vi "UHR-Fleezers Control (host) - Lorentz v5.vi"() -> ()   [LabVIEW 2014] (continued)
        n1320 = property on="Blue Laser ON" class="Bool (strict)"("Val(Sgnl)"="Blue Laser ON/OFF") -> ()  [unwired: 2 in, 2 out]
        n1321 = property on="Green Laser ON" class="Bool (strict)"("Val(Sgnl)"="Green Laser ON/OFF") -> ()  [unwired: 2 in, 2 out]
      }
      event "Laser interlacing mode", "Green Laser ON", "Red Laser ON", "Blue Laser ON": Value Change {
        n1322 = event-data() -> ()  [unwired: 7 out]
        n1323 = local write "Green Laser ON/OFF"("Green Laser ON") -> ()
        n1324 = local write "Blue Laser ON/OFF"("Blue Laser ON") -> ()
        n1325 = local write "Red Laser ON/OFF"("Red Laser ON") -> ()
        n1326 = case shown="False" "Green Laser ON" {
          tunnel: "Laser interlacing mode" -> [_ w2077]
          tunnel: [enum32{"Laser ON", "Laser OFF", "Interlace"}."Laser OFF" ("Green laser mode") w2077] -> w2053
          tunnel: [FALSE w2073] -> w2052
          frame False {
          }
          frame True {
            n1327 = local read "Green FB On/Off"() -> (w2074:bool)
            n1328 = Equal?(x=w2077, y=enum32{"Laser ON", "Laser OFF", "Interlace"}."Interlace") -> (x = y?=w2075:bool)
            n1329 = And(x=w2075, y=w2074) -> (x .and. y?=w2073:bool)
          }
        }
        n1330 = case shown="True" "Red Laser ON" {
          tunnel: "Laser interlacing mode" -> [_ w2070]
          tunnel: [enum32{"Laser ON", "Laser OFF", "Interlace"}."Laser OFF" ("Green laser mode") w2070] -> w2049
          tunnel: [FALSE w2066] -> w2048
          frame False {
          }
          frame True {
            n1331 = local read "Red FB On/Off"() -> (w2067:bool)
            n1332 = Equal?(x=w2070, y=enum32{"Laser ON", "Laser OFF", "Interlace"}."Interlace") -> (x = y?=w2068:bool)
            n1333 = And(x=w2068, y=w2067) -> (x .and. y?=w2066:bool)
          }
        }
        n1334 = case shown="True" "Blue Laser ON" {
          tunnel: "Laser interlacing mode" -> [_ w2061]
          tunnel: [enum32{"Laser ON", "Laser OFF", "Interlace"}."Laser OFF" ("Green laser mode") w2061] -> w2045
          tunnel: [FALSE w2059] -> w2044
          frame False {
          }
          frame True {
            n1335 = local read "Blue FB On/Off"() -> (w2060:bool)
            n1336 = Equal?(x=w2061, y=enum32{"Laser ON", "Laser OFF", "Interlace"}."Interlace") -> (x = y?=w2062:bool)
            n1337 = And(x=w2062, y=w2060) -> (x .and. y?=w2059:bool)
          }
        }
        n1338 = xnode "Read/Write Control"("FPGA VI Reference In"=w2043, "Operating Mode"=w2053, "Operating Mode 2"=w2053, "Green FB On/Off"=w2052, "Red Laser Operating Mode"=w2049, "RI Operating Mode 2"=w2049, "Red FB On/Off"=w2048, "BI Operating Mode (AO)"=w2045, "Blue Laser Operating Mode (D)"=w2045, "Blue FB On/Off"=w2044) -> ("error out"=w2054:errorcluster)  [unwired: 1 in, 1 out]
        n1339 = local read "Red FB On/Off"() -> (w2026:bool)
        n1340 = local read "Green FB On/Off"() -> (w2028:bool)
        n1341 = local read "Green Laser ON"() -> (w2027:bool)
        n1342 = local read "Red Laser ON"() -> (w2025:bool)
        n1343 = And(x=w2026, y=w2025) -> (x .and. y?=w2031:bool)
        n1344 = And(x=w2028, y=w2027) -> (x .and. y?=w2037:bool)
        n1345 = local read "Red laser intensity (V)"() -> (w2030:dbl)
        n1346 = local read "Red FB Setpoint (mV)"() -> (w2029:dbl)
        n1347 = local read "Green FB Setpoint (mV)"() -> (w2040:dbl)
        n1348 = local read "Green laser intensity (V)"() -> (w2042:dbl)
        n1349 = Multiply(x=w2030, y=1000.0) -> (x*y=w2034:dbl)
        n1350 = Subtract(x=w2029, y=5.0) -> (x-y=w2033:dbl)
        n1351 = Multiply(x=w2042, y=1000.0) -> (x*y=w2039:dbl)
        n1352 = Subtract(x=w2040, y=5.0) -> (x-y=w2038:dbl)
        n1353 = Less Or Equal?(x=w2034, y=w2033) -> (x <= y?=w2032:bool)
        n1354 = Less Or Equal?(x=w2039, y=w2038) -> (x <= y?=w2036:bool)
        n1355 = And(x=w2031, y=w2032) -> (x .and. y?=w2021:bool)
        n1356 = And(x=w2037, y=w2036) -> (x .and. y?=w2022:bool)
        n1357 = Or(x=w2022, y=w2021) -> (x .or. y?=w2020:bool)
        n1358 = case shown="True" w2020 {
          frame False {
            n1359 = local write "Laser Intensity Low (bugs to fix)"(FALSE ("Laser Intensity Low")) -> ()
          }
          frame True {
            n1360 = local write "Laser Intensity Low (bugs to fix)"(TRUE ("Laser Intensity Low")) -> ()
          }
        }
      }
      event "Invert laser interlacing": Value Change {
        n1361 = event-data() -> ()  [unwired: 7 out]
        n1362 = xnode "Read/Write Control"("FPGA VI Reference In"=w2078, "Invert GI"="Invert laser interlacing", "Invert GI 2"="Invert laser interlacing", "Invert RI"="Invert laser interlacing", "Invert RI 2"="Invert laser interlacing", "Invert BI (AO)"="Invert laser interlacing", "Invert BI (D)"="Invert laser interlacing") -> ("error out"=w2080:errorcluster)  [unwired: 1 in, 1 out]
      }
      event "Green FB Setpoint (mV)", "Green FB Gains", "Green FB On/Off", "Green Intensity % (FB OFF)", "Green int current ON count adj": Value Change {
        n1363 = event-data() -> ()  [unwired: 7 out]
        n1364 = local read "Green FB Setpoint (mV)"() -> (w2100:dbl)
        n1365 = Multiply(x=w2100, y=3.2767) -> (x*y=w2099:dbl)
        n1366 = local read "Green Intensity % (FB OFF)"() -> (w2103:dbl)
        n1367 = Multiply(x=w2103, y=655.35) -> (x*y=w2104:dbl)
        n1368 = To Unsigned Word Integer(number=w2104) -> (unsigned 16bit integer=w2102:u16)
        n1369 = local read "Green int current ON count adj"() -> (w2106:u32)
        n1370 = local read "Laser interlacing mode"() -> (w2097:enum32{"Laser ON", "Laser OFF", "Interlace"})
        n1371 = local read "Green FB Gains"() -> (w2094:T14)
        n1372 = local read "Green Laser ON"() -> (w2098:bool)
        n1373 = local read "Green FB On/Off"() -> (w2107:bool)
        n1374 = Equal?(x=w2097, y=enum32{"Laser ON", "Laser OFF", "Interlace"}."Interlace") -> (x = y?=w2095:bool)
        n1375 = Unbundle By Name(w2094) -> ("proportional gain (Kc)"=w2093:i16, "integral gain (Kc*Ts/Ti)"=w2092:i16, "derivative gain (Kc*Td/Ts)"=w2091:i16)
        n1376 = Compound Arithmetic op=AND(w2095, w2107, w2098) -> (w2081:bool)
        n1377 = local read "Green FB Setpoint (mV)"() -> (w2085:dbl)
        n1378 = local read "Green laser intensity (V)"() -> (w2088:dbl)
        n1379 = xnode "Read/Write Control"("FPGA VI Reference In"=w2090, "Green FB Setpoint"=w2099, "Green FB On/Off"=w2081, "Current Out"=w2102, "Green int current ON count adj"=w2106, "P3"=w2093, "I3"=w2092, "D3"=w2091) -> ("error out"=w2108:errorcluster)  [unwired: 1 in, 1 out]
        n1380 = Multiply(x=w2088, y=1000.0) -> (x*y=w2084:dbl)
        n1381 = Subtract(x=w2085, y=5.0) -> (x-y=w2083:dbl)
        n1382 = Less Or Equal?(x=w2084, y=w2083) -> (x <= y?=w2082:bool)
        n1383 = And(x=w2081, y=w2082) -> (x .and. y?=w2089:bool)
        n1384 = case shown="True" w2089 {
          frame False {
            n1385 = local write "Laser Intensity Low (bugs to fix)"(FALSE ("Laser Intensity Low")) -> ()
          }
          frame True {
            n1386 = local write "Laser Intensity Low (bugs to fix)"(TRUE ("Laser Intensity Low")) -> ()
          }
        }
      }
      event "Blue FB Setpoint (mV)", "Blue FB Gains", "Blue FB On/Off", "Blue Intensity % (FB OFF)", "Blue int AO ON count adjust": Value Change {
        # "Triggers blue laser serial command"
        # "16 bit analog out"
        n1387 = event-data() -> ()  [unwired: 7 out]
        n1388 = Multiply(x="Blue FB Setpoint (mV)", y=3.2767) -> (x*y=w2128:dbl)
        n1389 = Multiply(x="Blue Intensity % (FB OFF)", y=0.8) -> (x*y=w2111:dbl)
        n1390 = Number To Decimal String(number=w2111) -> (decimal integer string=w2112:string)  [unwired: 1 in]
        n1391 = Multiply(x="Blue Intensity % (FB OFF)", y=655.35) -> (x*y=w2131:dbl)
        n1392 = local write "Blue Laser Power (mW)\n(Constant Power Mode)"(w2112) -> ()
        n1393 = To Unsigned Word Integer(number=w2131) -> (unsigned 16bit integer=w2130:u16)
        n1394 = local read "Laser interlacing mode"() -> (w2126:enum32{"Laser ON", "Laser OFF", "Interlace"})
        n1395 = Unbundle By Name("Blue FB Gains") -> ("proportional gain (Kc)"=w2123:i16, "integral gain (Kc*Ts/Ti)"=w2122:i16, "derivative gain (Kc*Td/Ts)"=w2121:i16)
        n1396 = local read "Blue Laser ON"() -> (w2116:bool)
        n1397 = Equal?(x=w2126, y=enum32{"Laser ON", "Laser OFF", "Interlace"}."Interlace") -> (x = y?=w2124:bool)
        n1398 = Compound Arithmetic op=AND(w2124, "Blue FB On/Off", w2116) -> (w2127:bool)
        n1399 = xnode "Read/Write Control"("FPGA VI Reference In"=w2115, "Blue FB Setpoint"=w2128, "Blue FB On/Off"=w2127, "BI Current Out"=w2130, "Blue current ON count adj (AO)"="Blue int AO ON count adjust", "P5"=w2123, "I5"=w2122, "D5"=w2121) -> ("error out"=w2133:errorcluster)  [unwired: 1 in, 1 out]
      }
      event "Red FB Setpoint (mV)", "Red FB Gains", "Red FB On/Off", "Red Intensity % (FB OFF)": Value Change {
        n1400 = event-data() -> ()  [unwired: 7 out]
        n1401 = local read "Red FB Setpoint (mV)"() -> (w2154:dbl)
        n1402 = Multiply(x=w2154, y=3.2767) -> (x*y=w2153:dbl)
        n1403 = local read "Red Intensity % (FB OFF)"() -> (w2144:dbl)
        n1404 = Multiply(x=w2144, y=655.35) -> (x*y=w2157:dbl)
        n1405 = To Unsigned Word Integer(number=w2157) -> (unsigned 16bit integer=w2156:u16)
        n1406 = local read "Laser interlacing mode"() -> (w2151:enum32{"Laser ON", "Laser OFF", "Interlace"})
        n1407 = local read "Red FB Gains"() -> (w2148:T14)
        n1408 = local read "Red Laser ON"() -> (w2152:bool)
        n1409 = local read "Red FB On/Off"() -> (w2159:bool)
        n1410 = Equal?(x=w2151, y=enum32{"Laser ON", "Laser OFF", "Interlace"}."Interlace") -> (x = y?=w2149:bool)
        n1411 = Unbundle By Name(w2148) -> ("proportional gain (Kc)"=w2147:i16, "integral gain (Kc*Ts/Ti)"=w2146:i16, "derivative gain (Kc*Td/Ts)"=w2145:i16)
        n1412 = Compound Arithmetic op=AND(w2149, w2159, w2152) -> (w2136:bool)
        n1413 = local read "Red laser intensity (V)"() -> (w2135:dbl)
        n1414 = local read "Red FB Setpoint (mV)"() -> (w2134:dbl)
        n1415 = xnode "Read/Write Control"("FPGA VI Reference In"=w2143, "Red FB Setpoint"=w2153, "Red FB On/Off"=w2136, "RI Current Out"=w2156, "P4"=w2147, "I4"=w2146, "D4"=w2145) -> ("error out"=w2160:errorcluster)  [unwired: 1 in, 1 out]
        n1416 = Multiply(x=w2135, y=1000.0) -> (x*y=w2140:dbl)
        n1417 = Subtract(x=w2134, y=5.0) -> (x-y=w2139:dbl)
        n1418 = Less Or Equal?(x=w2140, y=w2139) -> (x <= y?=w2138:bool)
        n1419 = And(x=w2136, y=w2138) -> (x .and. y?=w2137:bool)
        n1420 = case shown="False" w2137 {
          frame False {
            n1421 = local write "Laser Intensity Low (bugs to fix)"(FALSE ("Laser Intensity Low")) -> ()
          }
          frame True {
            n1422 = local write "Laser Intensity Low (bugs to fix)"(TRUE ("Laser Intensity Low")) -> ()
          }
        }
      }
      event "+ phase (APD 1 Gate)", "- phase (APD 1 Gate)", "+ phase (APD 2 Gate)", "- phase (APD 2 Gate)", "+ phase (APD 3 Gate)", "- phase (APD 3 Gate)", "+ phase (APD Acq)", "- phase (APD Acq)": Value Change {
        n1423 = event-data() -> ()  [unwired: 7 out]
        n1424 = local read "Phase Adj. (APD 1 Gate)"() -> (w2183:i16)
        n1425 = Or(x="- phase (APD 1 Gate)", y="+ phase (APD 1 Gate)") -> (x .or. y?=w2185:bool)
        n1426 = Negate(x=w2183) -> (-x=w2190:i16)
        n1427 = Select(t=w2190, s="+ phase (APD 1 Gate)", f=w2183) -> (s? t:f=w2189:i16)
        n1428 = local read "Phase Adj. (APD 2 Gate)"() -> (w2180:i16)
        n1429 = Or(x="- phase (APD 2 Gate)", y="+ phase (APD 2 Gate)") -> (x .or. y?=w2178:bool)
        n1430 = Negate(x=w2180) -> (-x=w2182:i16)
        n1431 = Select(t=w2182, s="+ phase (APD 2 Gate)", f=w2180) -> (s? t:f=w2179:i16)
        n1432 = Negate(x="Phase Adj. (APD 3 Gate)") -> (-x=w2177:i16)
        n1433 = Or(x="- phase (APD 3 Gate)", y="+ phase (APD 3 Gate)") -> (x .or. y?=w2173:bool)
        n1434 = Select(t=w2177, s="+ phase (APD 3 Gate)", f="Phase Adj. (APD 3 Gate)") -> (s? t:f=w2174:i16)
        n1435 = local read "Phase Adj. (APD Acq)"() -> (w2171:i16)
        n1436 = Or(x="- phase (APD Acq)", y="+ phase (APD Acq)") -> (x .or. y?=w2169:bool)
        n1437 = Negate(x=w2171) -> (-x=w2172:i16)
        n1438 = Select(t=w2172, s="+ phase (APD Acq)", f=w2171) -> (s? t:f=w2170:i16)
        n1439 = xnode "Read/Write Control"("FPGA VI Reference In"=w2163, "Phase count adjustment (APD 1 Gate)"=w2189, "Phase count adjustment (APD 2 Gate)"=w2179, "Phase count adjustment (APD 3 Gate)"=w2174, "Phase Count Adjustment (APD Acq)"=w2170) -> ("FPGA VI Reference Out"=w2187:T35, "error out"=w2188:errorcluster)  [unwired: 1 in]
        n1440 = xnode "Read/Write Control"("FPGA VI Reference In"=w2187, "error in"=w2188, "+ phase (APD 1 Gate)"=w2185, "+ phase (APD 2 Gate)"=w2178, "+ phase (APD 3 Gate)"=w2173, "+ phase (APD Acq)"=w2169) -> ("error out"=w2186:errorcluster)  [unwired: 1 out]
      }
      event "Invert APD Gate", "APD Gate ON Count", "APD Gate OFF Count", "APD Gate", "APD Integration Time (s)", "APD AO Scale Factor", "Duty Frequency (ON 1/N cycles)", "Interlace ON count", "Interlace OFF count": Value Change {
        n1441 = event-data() -> ()  [unwired: 7 out]
        n1442 = Add(x="Interlace ON count", y="Interlace OFF count") -> (x+y=w2197:u16)
        n1443 = Add(x="APD Gate ON Count", y="APD Gate OFF Count") -> (x+y=w2208:u16)
        n1444 = Multiply(x="Duty Frequency (ON 1/N cycles)", y=w2197) -> (x*y=w2193:u16)
        "Green AI Count" <- w2193
        "Red AI Count" <- w2193
        "Blue AI Count" <- w2193
        n1445 = Subtract(x=w2193, y="Interlace ON count") -> (x-y=w2196:u16)
        n1446 = Multiply(x=w2208, y="Duty Frequency (ON 1/N cycles)") -> (x*y=w2207:u16)
        n1447 = Subtract(x=w2207, y="APD Gate ON Count") -> (x-y=w2206:u16)
        n1448 = local read "DMA Update Period (s)"() -> (w2209:dbl)
        n1449 = Multiply(x="APD Integration Time (s)", y=40000000.0) -> (x*y=w2213:dbl)
        n1450 = Reciprocal(x="APD Integration Time (s)") -> (1/x=→"APD Acq Rate (Hz)":dbl)
        n1451 = To Unsigned Long Integer(number=w2213) -> (unsigned 32bit integer=w2199:u32)
        "APD Int. Count" <- w2199
        n1452 = local read "Number of APDs"() -> (w2192:u8)
        n1453 = Divide(x=w2209, y="APD Integration Time (s)") -> (x/y=w2211:dbl)
        n1454 = Multiply(x=w2192, y=w2211) -> (x*y=w2210:dbl)
        n1455 = local write "APD Samples/FIFO Acq."(w2211) -> ()
        n1456 = local write "APD Elements/DMA read"(w2210) -> ()
        n1457 = xnode "Read/Write Control"("FPGA VI Reference In"=w2191, "Invert APD Gate"="Invert APD Gate", "APD Gate ON Count"="APD Gate ON Count", "APD Gate OFF Count"=w2206, "APD Acq Rate Count"=w2199, "APD Gate Operating Mode"="APD Gate", "APD AO scale factor"="APD AO Scale Factor", "Green interlace ON count"="Interlace ON count", "Green interlace OFF count"=w2196, "Green interlace ON count 2"="Interlace ON count", "Green interlace OFF count 2"=w2196, "Green FB Count"=w2193, "Red interlace ON count"="Interlace ON count", "Red interlace OFF count"="Interlace OFF count", "Blue ON count (AO)"="Interlace ON count", "Blue OFF count (AO)"="Interlace OFF count", "Blue interlace OFF count (D)"="Interlace OFF count", "Blue interlace ON count (D)"="Interlace ON count") -> ("error out"=w2215:errorcluster)  [unwired: 1 in, 1 out]
      }
      event "Neg. TTrig FPGA": Value Change {
        n1458 = event-data() -> ()  [unwired: 7 out]
        n1459 = xnode "Read/Write Control"("FPGA VI Reference In"=w2216, "TTrig Negate Pos"="Neg. TTrig FPGA") -> ()  [unwired: 1 in, 2 out]
      }
      event "Test ttrig": Value Change {
        n1460 = event-data() -> ()  [unwired: 7 out]
        n1461 = xnode "Read/Write Control"("FPGA VI Reference In"=w2218, "TTrig?"=TRUE) -> ("error out"=w2220:errorcluster)  [unwired: 1 in, 1 out]
      }
      event "Number of F/B Scans (AOD)", "Scan Speed (nm/s)", "Scan BD", "Initial delta (MHz)", "Step Size (nm)", "Scan Range (nm)": Value Change {
        w2284 = 123.0  # AOM cal (nm/MHz)
        n1462 = event-data() -> ()  [unwired: 7 out]
        n1463 = local read "BD 1 Frequency 1 (MHz)"() -> (w2267:dbl)
        n1464 = local read "AOM X Cal (nm/MHz)"() -> (w2259:dbl)
        n1465 = local read "X RF Frequency Limits (MHz)"() -> (w2271:T23)
        n1466 = local read "Y RF Frequency Limits (MHz)"() -> (w2268:T23)
        n1467 = local read "BD 2 Frequency 1 (MHz)"() -> (w2273:dbl)
        n1468 = Negate(x="Scan Range (nm)") -> (-x=w2237:dbl)
        n1469 = Divide(x=w2237, y=w2259) -> (x/y=w2241:dbl)
        n1470 = Select(t=w2271, s="Scan BD", f=w2268) -> (s? t:f=w2270:T23)
        n1471 = Select(t=w2267, s="Scan BD", f=w2273) -> (s? t:f=w2272:dbl)
        n1472 = Unbundle By Name(w2270) -> ("Maximum"=w2279:dbl, "Minimum"=w2278:dbl)
        n1473 = Add(x=w2241, y=w2272) -> (x+y=w2276:dbl)
        n1474 = Divide(x=w2237, y="Step Size (nm)") -> (x/y=w2256:dbl)
        n1475 = Divide(x="Step Size (nm)", y=w2259) -> (x/y=w2265:dbl)
        n1476 = Absolute Value(x=w2256) -> (abs(x)=w2240:dbl)
        n1477 = Sign(1:w2237) -> (0:w2238:dbl)
        n1478 = In Range and Coerce(upper limit=w2279, x=w2276, lower limit=w2278) -> (coerced(x)=w2275:dbl, In Range?=w2277:bool)
        n1479 = To Unsigned Quad Integer(1:w2240) -> (0:w2255:u64)
        "Scan steps (AOD)" <- w2255
        n1480 = call "IR AOM freq to word.vi"("Frequency In (MHz)"=w2265) -> ("Frequency Word Out (double)"=w2262:dbl)
        n1481 = Multiply(x=w2238, y=w2262) -> (x*y=w2239:dbl)
        n1482 = Subtract(x=w2276, y=w2275) -> (x-y=w2274:dbl)
        n1483 = To Quad Integer(1:w2239) -> (0:w2261:i64)
        "Incr. int (AOD)" <- w2261
        n1484 = Subtract(x=w2241, y=w2274) -> (x-y=w2260:dbl)
        "Scan Range (MHz)" <- w2260
        n1485 = Select(t=w2241, s=w2277, f=w2260) -> (s? t:f=w2280:dbl)
        n1486 = Multiply(x=w2260, y=w2259) -> (x*y=w2258:dbl)
        n1487 = Decrement(x=w2255) -> (x-1=w2308:u64)
        n1488 = Negate(x=w2258) -> (-x=w2254:dbl)
        n1489 = local write "Scan Range (nm)"(w2254) -> ()
        n1490 = Divide(x=w2280, y=w2308) -> (x/y=w2264:dbl)
        "Scan Increment (MHz)" <- w2264
        n1491 = call "IR AOM freq to word.vi"("Frequency In (MHz)"=w2264) -> ("Frequency Word Out (double)"=w2263:dbl)
        n1492 = Divide(x="Step Size (nm)", y="Scan Speed (nm/s)") -> (x/y=w2251:dbl)
        n1493 = To Quad Integer(1:w2263) -> ()  [unwired: 1 out]
        n1494 = local read "Number Interlace Sets"() -> (w2235:u8)
        n1495 = local read "AI Count (ticks)"() -> (w2236:u16)
        n1496 = local read "Total Counts (ticks)"() -> (w2234:u16)
        n1497 = local read "# Samples/trap"() -> (w2266:u32)
        n1498 = Multiply(x=w2236, y=w2235) -> (x*y=w2233:u16)
        n1499 = Divide(x=w2234, y=w2233) -> (x/y=w2232:dbl)
        n1500 = Select(t=w2267, s="Scan BD", f=w2273) -> (s? t:f=w2305:dbl)
        "Initial freq. (MHz)" <- w2305
        n1501 = Add(x=w2280, y=w2305) -> (x+y=→"Final freq. (MHz)":dbl)
        n1502 = Divide(x=w2234, y=40000000.0) -> (x/y=w2250:dbl)
        n1503 = Divide(x=w2251, y=w2250) -> (x/y=w2249:dbl)
        n1504 = To Unsigned Quad Integer(1:w2249) -> (0:w2224:u64)
        n1505 = Quotient & Remainder(x=w2224, y=u64 2) -> (x-y*floor(x/y)=w2228:u64)  [unwired: 1 out]
        n1506 = Equal?(x=w2228, y=u64 0) -> (x = y?=w2226:bool)
        n1507 = Decrement(x=w2224) -> (x-1=w2225:u64)
        n1508 = Select(t=w2224, s=w2226, f=w2225) -> (s? t:f=w2223:u64)
        "Cycles/step (AOD)" <- w2223
        n1509 = xnode "Read/Write Control"("FPGA VI Reference In"=w2222, "Scan steps"=w2255, "Number of scans"="Number of F/B Scans (AOD)", "Cycles per step"=w2223, "Scan freq.  increment"=w2261, "Scan BD"="Scan BD") -> ("error out"=w2314:errorcluster)  [unwired: 1 in, 1 out]
        n1510 = Multiply(x=w2255, y=w2223) -> (x*y=w2309:u64)
        n1511 = Multiply(x=w2309, y=u64 2) -> (x*y=w2231:u64)
        n1512 = Multiply(x=w2232, y=w2231) -> (x*y=w2230:dbl)
        "Data points/scan (f/b)" <- w2230
        n1513 = Multiply(x=w2230, y="Number of F/B Scans (AOD)") -> (x*y=w2312:dbl)
        "Data points/scans" <- w2312
        n1514 = Divide(x=w2312, y=w2266) -> (x/y=→"N sets should be saved":dbl)
        n1515 = Multiply(x=w2309, y=w2250) -> (x*y=w2248:dbl)
        "Time/Scan (s) (AOD)" <- w2248
        n1516 = Select(t=w2280, s="Scan BD", f=0.0) -> (s? t:f=w2306:dbl)
        n1517 = Select(t=0.0, s="Scan BD", f=w2280) -> (s? t:f=w2302:dbl)
        n1518 = local read "BD 2 Frequency 2 (MHz)"() -> (w2298:dbl)
        n1519 = local read "BD 1 Frequency 2 (MHz)"() -> (w2301:dbl)
        n1520 = Add(x=w2302, y=w2273) -> (x+y=w2299:dbl)
        n1521 = Add(x=w2267, y=w2306) -> (x+y=w2300:dbl)
        n1522 = Multiply(x=w2248, y=2.0) -> (x*y=w2247:dbl)
        n1523 = Multiply(x=w2247, y="Number of F/B Scans (AOD)") -> (x*y=w2244:dbl)
        n1524 = Divide(x=w2244, y=60.0) -> (x/y=→"Time to Finish All (min)":dbl)
        n1525 = Add(x="Trap 2 Bead Size (nm)", y="Trap 1 Bead Size (nm)") -> (x+y=w2288:dbl)
        n1526 = Divide(x=w2288, y=2.0) -> (x/y=w2282:dbl)
        n1527 = local read "Initial delta (MHz)"() -> (w2285:dbl)
        n1528 = Subtract(x=w2299, y=w2298) -> (x-y=w2296:dbl)
        n1529 = Subtract(x=w2300, y=w2301) -> (x-y=w2297:dbl)
        n1530 = Square(x=w2296) -> (x^2=w2295:dbl)
        n1531 = Square(x=w2297) -> (x^2=w2294:dbl)
        n1532 = Add(x=w2294, y=w2295) -> (x+y=w2293:dbl)
        n1533 = Square Root(x=w2293) -> (sqrt(x)=w2292:dbl)
        "Final delta (MHz)" <- w2292
        n1534 = Multiply(x=w2284, y=w2292) -> (x*y=w2291:dbl)
        n1535 = Multiply(x=w2285, y=w2284) -> (x*y=w2283:dbl)
        n1536 = Subtract(x=w2283, y=w2282) -> (x-y=→"Initial sep (nm)":dbl)
        n1537 = Subtract(x=w2291, y=w2282) -> (x-y=→"Final sep (nm)":dbl)
      }
      event "Freq or Amp switch first", "Swap F1 and F2", "Freq switch delay", "Amp switch delay": Value Change {
        n1538 = event-data() -> ()  [unwired: 7 out]
        n1539 = local read "Amp switch delay"() -> (w2316:u16)
        n1540 = local read "Swap F1 and F2"() -> (w2317:bool)
        n1541 = xnode "Read/Write Control"("FPGA VI Reference In"=w2315, "Swap F1 and F2"=w2317, "Amp switch delay"=w2316) -> ("error out"=w2318:errorcluster)  [unwired: 1 in, 1 out]
      }
      event "Scan steps (MCL)", "Number of scans (MCL)", "Scan Range (V)\n(of steps)", "2D or 1D Scan", "N APD Samp/step", "Fast Scan Dir", "Continuous MCL Scanning", "Scan lines (y)": Value Change {
        w2321 = 32767.0 ("y")
        n1542 = event-data() -> ()  [unwired: 7 out]
        n1543 = Select(t="Scan lines (y)", s="2D or 1D Scan", f="Number of scans (MCL)") -> (s? t:f=w2326:u64)
        n1544 = Decrement(x="Scan steps (MCL)") -> (x-1=w2342:u64)
        n1545 = Divide(x="Scan Range (V)\n(of steps)", y=w2342) -> (x/y=w2341:dbl)
        "Desired Scan Incr (V)" <- w2341
        n1546 = local read "APD Integration Time (s)"() -> (w2334:dbl)
        n1547 = Multiply(x=w2341, y=w2321) -> (x*y=w2350:dbl)
        n1548 = Divide(x=w2350, y=10.0) -> (x/y=w2340:dbl)
        "Desired incr (int)" <- w2340
        n1549 = local read "Update Count (MCL)"() -> (w2346:u32)
        n1550 = Round Toward -Infinity(1:w2340) -> (0:w2349:dbl)
        n1551 = To Word Integer(number=w2349) -> (16bit integer=w2324:i16)
        "Actual Incr. int (MCL)" <- w2324
        n1552 = Multiply(x=w2334, y=40000000.0) -> (x*y=w2347:dbl)
        n1553 = Divide(x=w2347, y=w2346) -> (x/y=w2345:dbl)
        n1554 = Multiply(x=i16 10, y=w2324) -> (x*y=w2322:i16)
        n1555 = Multiply(x="N APD Samp/step", y=w2345) -> (x*y=w2344:dbl)
        "Cycles/step (MCL)" <- w2344
        n1556 = Divide(x=w2322, y=w2321) -> (x/y=→"Actual MCL Inc (V)":dbl)
        n1557 = Multiply(x="N APD Samp/step", y="Scan steps (MCL)") -> (x*y=w2336:dbl)
        n1558 = local read "APD Samples/FIFO Acq."() -> (w2333:dbl)
        n1559 = Multiply(x=w2336, y=u64 2) -> (x*y=w2335:dbl)
        "Data points/scan (f+b)" <- w2335
        n1560 = Multiply(x=w2335, y=w2326) -> (x*y=w2353:dbl)
        "Data points/scans (MCL)" <- w2353
        n1561 = Multiply(x=w2334, y=w2335) -> (x*y=w2327:dbl)
        "Time/f+b scan (s) (MCL)" <- w2327
        n1562 = Divide(x=w2353, y=w2333) -> (x/y=→"N sets should be saved (MCL)":dbl)
        n1563 = Multiply(x=w2327, y=w2326) -> (x*y=→"Total Time (s)":dbl)
        n1564 = Not(x="Fast Scan Dir") -> (.not. x?=w2331:bool)
        n1565 = xnode "Read/Write Control"("FPGA VI Reference In"=w2319, "Scan steps (MCL)"="Scan steps (MCL)", "Number of scans (MCL)"=w2326, "Cycles per step (MCL)"=w2344, "Scan freq.  increment (MCL)"=w2324, "1D or 2D Scan?"="2D or 1D Scan", "MCL Scan Axis"=w2331, "Cont. Scan (MCL)"="Continuous MCL Scanning") -> ("error out"=w2355:errorcluster)  [unwired: 1 in, 1 out]
      }
      event "Read Cal": Value Change {
        w2394 = 1000.0 ("y")
        w2377 = T44."big-endian, network order" ("byte order (0:big-endian, network order)")
        w2378 = -1 ("count (1)")
        n1566 = event-data() -> ()  [unwired: 7 out]
        n1567 = local read "Save file name"() -> (w2410:path)
        n1568 = local write "Read Cal"(FALSE ("Read Cal")) -> ()
        n1569 = Strip Path(path=w2410) -> (stripped path=w2409:path)  [unwired: 1 out]
        n1570 = Path To String(path=w2409) -> (string=w2386:string)
        n1571 = Concatenate Strings(w2386, "\\current.cal" ("string")) -> (w2407:string)
        n1572 = Concatenate Strings(w2386, "\\current.off" ("string")) -> (w2384:string)
        n1573 = String To Path(string=w2407) -> (path=w2406:path)
        n1574 = String To Path(string=w2384) -> (path=w2381:path)
        n1575 = Open/Create/Replace File(file path (use dialog)=w2406, operation (0:open)=T43."open", access (0:read/write)=enum16{"read/write", "read-only", "write-only"}."read-only") -> (refnum out=w2413:refnum<file>, error out=w2402:errorcluster)  [unwired: 1 in, 3 out]
        n1576 = Open/Create/Replace File(file path (use dialog)=w2381, operation (0:open)=T43."open", access (0:read/write)=enum16{"read/write", "read-only", "write-only"}."read-only") -> (refnum out=w2380:refnum<file>)  [unwired: 1 in, 4 out]
        n1577 = Deny Access(4:w2402, 7:w2413) -> (0:w2401:errorcluster, 3:w2405:refnum<file>)  [unwired: 1 out]
        n1578 = Deny Access(7:w2380) -> (3:w2379:refnum<file>)  [unwired: 1 in, 2 out]
        n1579 = Read from Binary File(5:0.0, 8:w2401, 9:w2377, 10:w2378, 11:w2405) -> (0:w2400:errorcluster, 2:w2398:dbl[], 3:w2403:refnum<file>)  [unwired: 2 out]
        n1580 = Array To Cluster(array=w2398) -> (cluster=w2397:T46)
        n1581 = Unbundle(w2397) -> ("[0]"=w2365:dbl, "[1]"=w2363:dbl, "[2]"=w2364:dbl, "[3]"=w2362:dbl, "[4]"=w2396:dbl, "[5]"=w2395:dbl)
        n1582 = Close File(refnum=w2403, error in=w2400) -> (error out=→"Read cal error":errorcluster)  [unwired: 1 out]
        n1583 = Multiply(x=w2396, y=w2394) -> (x*y=w2391:dbl)
        n1584 = Multiply(x=w2395, y=w2394) -> (x*y=w2387:dbl)
        n1585 = Read from Binary File(5:0.0, 9:w2377, 10:w2378, 11:w2379) -> (2:w2373:dbl[], 3:w2371:refnum<file>)  [unwired: 1 in, 3 out]
        n1586 = Close File(refnum=w2371) -> ()  [unwired: 1 in, 2 out]
        n1587 = Bundle By Name(cluster="T1 calibration", "T1 alpha_x (nm/V)"=w2365, "T1 offset_x (mV)"=w2391, "T1 kappa_x (pN/nm)"=w2364) -> (w2390:T9)
        n1588 = Array Subset(array=w2373, index=1) -> (w2370:dbl[])  [unwired: 1 in]
        n1589 = Bundle By Name(cluster="T2 calibration", "T2 alpha_x (nm/V)"=w2363, "T2 offset_x (mV)"=w2387, "T2 kappa_x (pN/nm)"=w2362) -> (w2388:T8)
        n1590 = Index Array(array=w2373, index=0) -> (element=→"Offset file step size":dbl)
        n1591 = local write "T1 calibration"(w2390) -> ()
        n1592 = local write "T2 calibration"(w2388) -> ()
        n1593 = Decimate 1D Array(w2370) -> (w2360:dbl[], w2359:dbl[])  [unwired: 1 out]
        n1594 = Multiply(x=w2365, y=w2364) -> (x*y=w2366:dbl)
        n1595 = Multiply(x=w2363, y=w2362) -> (x*y=w2367:dbl)
        n1596 = Divide(x=w2367, y=w2366) -> (x/y=w2358:dbl)
        n1597 = property on="B factor" class="DigNum (strict)"("Val(Sgnl)"=w2358) -> ()  [unwired: 2 in, 2 out]
        n1598 = Bundle By Name(cluster="Offset Values", "Trap 1X offset"=w2360, "Trap 2X offset"=w2359) -> (w2368:T20)
        n1599 = Multiply(x=w2359, y=w2358) -> (x*y=w2361:dbl[])
        n1600 = local write "Offset Values"(w2368) -> ()
        n1601 = Subtract(x=w2360, y=w2361) -> (x-y=w2356:dbl[])
        n1602 = case shown="True" "Auto read offset correction" {
          tunnel: w2356 -> [_ w2414]
          frame False {
          }
          frame True {
            n1603 = property on="Setpoint offset\ncorrection values" class="Arr (strict)"("Val(Sgnl)"=w2414) -> ()  [unwired: 2 in, 2 out]
          }
        }
      }
      event "Abort MCL Scan": Value Change {
        n1604 = event-data() -> ()  [unwired: 7 out]
        n1605 = local write "MCL Scanning"(FALSE ("MCL Scanning")) -> ()
        n1606 = xnode "Read/Write Control"("FPGA VI Reference In"=w2415, "Abort scan (MCL)"="Abort MCL Scan") -> ("error out"=w2418:errorcluster)  [unwired: 1 in, 1 out]
      }
      event "Update Count (MCL)": Value Change {
        n1607 = event-data() -> ()  [unwired: 7 out]
        n1608 = xnode "Read/Write Control"("FPGA VI Reference In"=w2419, "MCL count"="Update Count (MCL)") -> ("error out"=w2421:errorcluster)  [unwired: 1 in, 1 out]
      }
      event "+ phase (MCL)", "- phase (MCL)": Value Change {
        n1609 = event-data() -> ()  [unwired: 7 out]
        n1610 = Or(x="- phase (MCL)", y="+ phase (MCL)") -> (x .or. y?=w2425:bool)
        n1611 = Negate(x="Phase adjust (MCL)") -> (-x=w2431:i16)
        n1612 = Select(t=w2431, s="+ phase (MCL)", f="Phase adjust (MCL)") -> (s? t:f=w2429:i16)
        n1613 = xnode "Read/Write Control"("FPGA VI Reference In"=w2422, "Phase count adjustment (MCL)"=w2429) -> ("FPGA VI Reference Out"=w2426:T35, "error out"=w2427:errorcluster)  [unwired: 1 in]
        n1614 = xnode "Read/Write Control"("FPGA VI Reference In"=w2426, "error in"=w2427, "+ phase (MCL)"=w2425) -> ("error out"=w2424:errorcluster)  [unwired: 1 out]
      }
      event "Abort AOD Scan": Value Change {
        n1615 = event-data() -> ()  [unwired: 7 out]
        n1616 = xnode "Read/Write Control"("FPGA VI Reference In"=w2432, "Abort scan"="Abort AOD Scan") -> ("error out"=w2434:errorcluster)  [unwired: 1 in, 1 out]
      }
      event "Continuous AOD Scanning": Value Change {
        n1617 = event-data() -> ()  [unwired: 7 out]
        n1618 = xnode "Read/Write Control"("FPGA VI Reference In"=w2435, "Cont. Scan"="Continuous AOD Scanning") -> ("error out"=w2437:errorcluster)  [unwired: 1 in, 1 out]
      }
      event "Index": Value Change {
        n1619 = event-data() -> ()  [unwired: 7 out]
        n1620 = call "Create new save file.vi"("Insert"="", "Ext"=".dat" ("string"), "Index In"="Index") -> ("Path Out"=→"Save file name":path, "Index Out"=w2438:dbl)
        "Save index" <- w2438
        n1621 = local write "Index"(w2438) -> ()
      }
      event "AO1", "AO2": Value Change {
        w2452 = 10.0 ("y")
        w2451 = 32767.0 ("y")
        n1622 = event-data() -> ()  [unwired: 7 out]
        n1623 = local read "AO2"() -> (w2450:dbl)
        n1624 = local read "AO1"() -> (w2447:dbl)
        n1625 = Multiply(x=w2447, y=w2451) -> (x*y=w2446:dbl)
        n1626 = Multiply(x=w2450, y=w2451) -> (x*y=w2449:dbl)
        n1627 = Divide(x=w2446, y=w2452) -> (x/y=w2445:dbl)
        n1628 = Divide(x=w2449, y=w2452) -> (x/y=w2448:dbl)
        n1629 = To Word Integer(number=w2445) -> (16bit integer=w2453:i16)
        n1630 = To Word Integer(number=w2448) -> (16bit integer=w2454:i16)
        n1631 = xnode "Read/Write Control"("FPGA VI Reference In"=w2443, "AO1"=w2453, "AO2"=w2454) -> ("error out"=w2444:errorcluster)  [unwired: 1 in, 1 out]
      }
      event "Inject Pump 1": Value Change {
        n1632 = event-data() -> ()  [unwired: 7 out]
        n1633 = disable-structure shown="Disabled" {
          disable-tunnel: w2455 -> [w2456 _]
          frame Disabled {
            n1634 = local read "Use Harvard pumps\nfor beads (else Chemyx)"() -> (w2457:bool)
            n1635 = case shown="True" w2457 {
              tunnel: "Inject Pump 1" -> [w2461 w2502]
              tunnel: w2456 -> [_ w2503]
              frame False {
                n1636 = local read "Pump write delay (ms)"() -> (w2460:dbl)
                n1637 = local read "Chemyx Syringe Pump Serial Port"() -> (w2459:refnum<visa-resource-name>)
                n1638 = case shown="True" w2461 {
                  tunnel: w2460 -> [w2467 w2481]
                  tunnel: w2459 -> [w2464 w2480]
                  frame False {
                    n1639 = flat-sequence {
                      tunnel: w2464 -> [w2468]
                      tunnel: [w2468] -> w2465
                      tunnel: w2467 -> [_]
                      tunnel: [w2471] -> w2466
                      tunnel: w2465 -> [w2471]
                      tunnel: w2466 -> [w2472]
                      tunnel: [w2472] -> w2462
                      tunnel: [w2474] -> w2463
                      tunnel: w2462 -> [w2474]
                      tunnel: w2463 -> [w2476]
                      frame #0 {
                        n1640 = call "Write to pump.vi"("string"="enter pump1", "VISA resource name"=w2468) -> ()  [unwired: 1 out]
                      }
                      frame #1 {
                        n1641 = Wait (ms)(milliseconds to wait="Pump pause delay (ms)") -> ()  [unwired: 1 out]
                      }
                      frame #2 {
                        n1642 = call "Write to pump.vi"("string"="stop", "VISA resource name"=w2472) -> ()  [unwired: 1 out]
                      }
                      frame #3 {
                        n1643 = Wait (ms)(milliseconds to wait=u32 500) -> ()  [unwired: 1 out]
                      }
                      frame #4 {
                        n1644 = call "Write to pump.vi"("string"="stop", "VISA resource name"=w2476) -> ()  [unwired: 1 out]
                      }
                    }
                  }
                  frame True {
                    n1645 = flat-sequence {
                      tunnel: w2480 -> [w2490]
                      tunnel: w2481 -> [w2485]
                      tunnel: w2481 -> [w2492]
                      tunnel: w2480 -> [w2493]
                      tunnel: [w2493] -> w2478
                      tunnel: [w2495] -> w2479
                      tunnel: w2478 -> [w2495]
                      tunnel: w2479 -> [w2497]
                      frame #0 {
                        n1646 = local read "All Pump Parameters"() -> (w2484:T10)
                        n1647 = Unbundle By Name(w2484) -> ("Pump 1"=w2491:T47)
                        n1648 = call "Set pump parameters.vi"("Pump write delay (ms)"=w2485, "Volume (uL)"="Ch 1 Inject Volume (uL)", "Rate (uL/h)"="Ch 1 Inject Rate (ul/h)", "Units"=4.0, "Pump #"=1.0, "Pump Parameters In"=w2491, "VISA resource name"=w2490) -> ("Pump Parameters Out"=w2483:T47)  [unwired: 3 in]
                        n1649 = Bundle By Name(cluster=w2484, "Pump 1"=w2483) -> (w2482:T10)
                        n1650 = local write "All Pump Parameters"(w2482) -> ()
                      }
                      frame #1 {
                        n1651 = Wait (ms)(milliseconds to wait=w2492) -> ()  [unwired: 1 out]
                      }
                      frame #2 {
                        n1652 = call "Write to pump.vi"("string"="start", "VISA resource name"=w2493) -> ()  [unwired: 1 out]
                      }
                      frame #3 {
                        n1653 = Wait (ms)(milliseconds to wait=u32 500) -> ()  [unwired: 1 out]
                      }
                      frame #4 {
                        n1654 = call "Write to pump.vi"("string"="start", "VISA resource name"=w2497) -> ()  [unwired: 1 out]
                      }
                    }
                  }
                }
              }
              frame True {
                n1655 = case shown="False" w2502 {
                  tunnel: w2503 -> [w2515 w2525]
                  frame False {
                    n1656 = flat-sequence {
                      tunnel: w2515 -> [w2517]
                      frame #0 {
                        n1657 = local write "Flushing P1"(FALSE ("Flushing P1")) -> ()
                        n1658 = Concatenate Strings("stop" ("string"), "\r") -> (w2519:string)
                        n1659 = VISA Write(VISA resource name=w2517, write buffer=w2519) -> ()  [unwired: 1 in, 3 out]
                      }
                      frame #1 {
                        n1660 = property on="Clear Volume P1" class="Bool (strict)"("Val(Sgnl)"=TRUE ("Value (Signaling)")) -> ()  [unwired: 2 in, 2 out]
                      }
                    }
                  }
                  frame True {
                    n1661 = local read "Normal Flow Rate (ul/h) P1"() -> (w2523:dbl)
                    n1662 = Number To Decimal String(number=w2523) -> (decimal integer string=w2529:string)  [unwired: 1 in]
                    n1663 = Concatenate Strings("irate  " ("string"), w2529, " u/h" ("string"), "\r") -> (w2527:string)
                    n1664 = VISA Write(VISA resource name=w2525, write buffer=w2527) -> (VISA resource name out=w2524:refnum<visa-resource-name>)  [unwired: 1 in, 2 out]
                    n1665 = Concatenate Strings("irun" ("string"), "\r") -> (w2531:string)
                    n1666 = VISA Write(VISA resource name=w2524, write buffer=w2531) -> ()  [unwired: 1 in, 3 out]
                  }
                }
                n1667 = local read "Saving..."() -> (w2500:bool)
                n1668 = local read "Save Event Log?"() -> (w2499:bool)
                n1669 = And(x=w2500, y=w2499) -> (x .and. y?=w2501:bool)
                n1670 = case shown="True" w2501 {
                  tunnel: w2502 -> [_ w2513]
                  frame False {
                  }
                  frame True {
                    n1671 = local read "Normal Flow Rate (ul/h) P1"() -> (w2504:dbl)
                    n1672 = Number To Decimal String(number=w2504) -> (decimal integer string=w2505:string)  [unwired: 1 in]
                    n1673 = Concatenate Strings("on, flow rate", w2505) -> (w2507:string)
                    n1674 = Select(t=w2507, s=w2513, f="off") -> (s? t:f=w2509:string)
                    n1675 = local read "log file ref"() -> (w2514:refnum<file>)
                    n1676 = local read "Time (s)"() -> (w2508:dbl)
                    n1677 = Concatenate Strings("pump 1 ", w2509) -> (w2511:string)
                    n1678 = call "write to event log.vi"("log file ref"=w2514, "time"=w2508, "input string"=w2511) -> ()  [unwired: 8 in]
                  }
                }
              }
            }
          }
          frame Enabled {
          }
        }
      }
      event "Shunt 1": Value Change {
        n1679 = event-data() -> ()  [unwired: 7 out]
        n1680 = local read "Visa resource for valves"() -> (w2533:refnum<visa-resource-name>)
        n1681 = call "hamilton_controller.vi"("VISA resource name in"=w2533, "Open?"="Shunt 1", "valve"=enum16{"A", "B", "ALL"}."A", "action"=T41."MOVE VALVE") -> ("error out"=w2535:errorcluster)  [unwired: 6 in, 1 out]
      }
      event "Shunt 2": Value Change {
        n1682 = event-data() -> ()  [unwired: 7 out]
        n1683 = local read "Visa resource for valves"() -> (w2538:refnum<visa-resource-name>)
        n1684 = call "hamilton_controller.vi"("VISA resource name in"=w2538, "Open?"="Shunt 2", "valve"=enum16{"A", "B", "ALL"}."B", "action"=T41."MOVE VALVE") -> ("error out"=w2539:errorcluster)  [unwired: 6 in, 1 out]
      }
      event "Inject Pump 3": Value Change {
        n1685 = event-data() -> ()  [unwired: 7 out]
        n1686 = local read "Use Harvard pumps\nfor beads (else Chemyx)"() -> (w2544:bool)
        n1687 = disable-structure shown="Disabled" {
          disable-tunnel: w2544 -> [w2546 _]
          disable-tunnel: w2543 -> [w2545 _]
          frame Disabled {
            n1688 = case shown="True" w2546 {
              tunnel: "Inject Pump 3" -> [w2550 w2591]
              tunnel: w2545 -> [_ w2592]
              frame False {
                n1689 = local read "Pump write delay (ms)"() -> (w2549:dbl)
                n1690 = case shown="True" w2550 {
                  tunnel: w2549 -> [w2556 w2570]
                  tunnel: "Chemyx Syringe Pump Serial Port" -> [w2553 w2569]
                  frame False {
                    n1691 = flat-sequence {
                      tunnel: w2553 -> [w2557]
                      tunnel: [w2557] -> w2554
                      tunnel: w2556 -> [_]
                      tunnel: [w2560] -> w2555
                      tunnel: w2554 -> [w2560]
                      tunnel: w2555 -> [w2561]
                      tunnel: [w2561] -> w2551
                      tunnel: [w2563] -> w2552
                      tunnel: w2551 -> [w2563]
                      tunnel: w2552 -> [w2565]
                      frame #0 {
                        n1692 = call "Write to pump.vi"("string"="enter pump3", "VISA resource name"=w2557) -> ()  [unwired: 1 out]
                      }
                      frame #1 {
                        n1693 = local read "Pump pause delay (ms)"() -> (w2559:u32)
                        n1694 = Wait (ms)(milliseconds to wait=w2559) -> ()  [unwired: 1 out]
                      }
                      frame #2 {
                        n1695 = call "Write to pump.vi"("string"="stop", "VISA resource name"=w2561) -> ()  [unwired: 1 out]
                      }
                      frame #3 {
                        n1696 = Wait (ms)(milliseconds to wait=u32 0) -> ()  [unwired: 1 out]
                      }
                      frame #4 {
                        n1697 = call "Write to pump.vi"("string"="stop", "VISA resource name"=w2565) -> ()  [unwired: 1 out]
                      }
                    }
                  }
                  frame True {
                    n1698 = flat-sequence {
                      tunnel: w2569 -> [w2579]
                      tunnel: w2570 -> [w2574]
                      tunnel: w2570 -> [w2581]
                      tunnel: w2569 -> [w2582]
                      tunnel: [w2582] -> w2568
                      tunnel: [w2585] -> w2567
                      tunnel: w2568 -> [w2585]
                      tunnel: w2567 -> [w2586]
                      frame #0 {
                        n1699 = local read "All Pump Parameters"() -> (w2573:T10)
                        n1700 = Unbundle By Name(w2573) -> ("Pump 3"=w2580:T47)
                        n1701 = call "Set pump parameters.vi"("Pump write delay (ms)"=w2574, "Volume (uL)"="Ch 3 Inject Volume (uL)", "Rate (uL/h)"="Ch 3 Inject Rate (ul/h)", "Units"=4.0, "Pump #"=3.0, "Pump Parameters In"=w2580, "VISA resource name"=w2579) -> ("Pump Parameters Out"=w2572:T47)  [unwired: 3 in]
                        n1702 = Bundle By Name(cluster=w2573, "Pump 3"=w2572) -> (w2571:T10)
                        n1703 = local write "All Pump Parameters"(w2571) -> ()
                      }
                      frame #1 {
                        n1704 = Wait (ms)(milliseconds to wait=w2581) -> ()  [unwired: 1 out]
                      }
                      frame #2 {
                        n1705 = call "Write to pump.vi"("string"="start", "VISA resource name"=w2582) -> ()  [unwired: 1 out]
                      }
                      frame #3 {
                        n1706 = Wait (ms)(milliseconds to wait=u32 500) -> ()  [unwired: 1 out]
                      }
                      frame #4 {
                        n1707 = call "Write to pump.vi"("string"="start", "VISA resource name"=w2586) -> ()  [unwired: 1 out]
                      }
                    }
                  }
                }
              }
              frame True {
                n1708 = case shown="False" w2591 {
                  tunnel: w2592 -> [w2604 w2611]
                  frame False {
                    n1709 = flat-sequence {
                      tunnel: w2604 -> [w2606]
                      frame #0 {
                        n1710 = local write "Flushing P3"(FALSE ("Flushing P3")) -> ()
                        n1711 = Concatenate Strings("stop" ("string"), "\r") -> (w2608:string)
                        n1712 = VISA Write(VISA resource name=w2606, write buffer=w2608) -> ()  [unwired: 1 in, 3 out]
                      }
                      frame #1 {
                        n1713 = property on="Clear Volume P3" class="Bool (strict)"("Val(Sgnl)"=TRUE ("Value (Signaling)")) -> ()  [unwired: 2 in, 2 out]
                      }
                    }
                  }
                  frame True {
                    n1714 = local read "Normal Flow Rate (ul/h) P3"() -> (w2612:dbl)
                    n1715 = Number To Decimal String(number=w2612) -> (decimal integer string=w2618:string)  [unwired: 1 in]
                    n1716 = Concatenate Strings("irate  " ("string"), w2618, " u/h" ("string"), "\r") -> (w2616:string)
                    n1717 = VISA Write(VISA resource name=w2611, write buffer=w2616) -> (VISA resource name out=w2614:refnum<visa-resource-name>)  [unwired: 1 in, 2 out]
                    n1718 = Concatenate Strings("irun" ("string"), "\r") -> (w2620:string)
                    n1719 = VISA Write(VISA resource name=w2614, write buffer=w2620) -> ()  [unwired: 1 in, 3 out]
                  }
                }
                n1720 = local read "Save Event Log?"() -> (w2589:bool)
                n1721 = local read "Saving..."() -> (w2590:bool)
                n1722 = And(x=w2590, y=w2589) -> (x .and. y?=w2588:bool)
                n1723 = case shown="True" w2588 {
                  tunnel: w2591 -> [_ w2599]
                  frame False {
                  }
                  frame True {
                    n1724 = local read "Normal Flow Rate (ul/h) P3"() -> (w2593:dbl)
                    n1725 = Number To Decimal String(number=w2593) -> (decimal integer string=w2595:string)  [unwired: 1 in]
                    n1726 = Concatenate Strings("on, flow rate", w2595) -> (w2594:string)
                    n1727 = local read "log file ref"() -> (w2598:refnum<file>)
                    n1728 = Select(t=w2594, s=w2599, f="off") -> (s? t:f=w2600:string)
                    n1729 = local read "Time (s)"() -> (w2597:dbl)
                    n1730 = Concatenate Strings("pump 3 ", w2600) -> (w2602:string)
                    n1731 = call "write to event log.vi"("log file ref"=w2598, "time"=w2597, "input string"=w2602) -> ()  [unwired: 8 in]
                  }
                }
              }
            }
          }
          frame Enabled {
          }
        }
      }
      event "Inject Pump 2": Value Change {
        n1732 = event-data() -> ()  [unwired: 7 out]
        n1733 = local read "Pump write delay (ms)"() -> (w2627:dbl)
        n1734 = local read "Chemyx Syringe Pump Serial Port"() -> (w2626:refnum<visa-resource-name>)
        n1735 = flat-sequence {
          tunnel: w2626 -> [w2651]
          tunnel: w2627 -> [w2647]
          tunnel: "Inject Pump 2" -> [_]
          tunnel: w2627 -> [w2653]
          tunnel: w2626 -> [w2654]
          frame #0 {
            n1736 = local read "All Pump Parameters"() -> (w2646:T10)
            n1737 = Multiply(x=60.0, y="Flush Center Ch Rate (ul/m)") -> (x*y=w2643:dbl)
            n1738 = Unbundle By Name(w2646) -> ("Pump 2"=w2652:T47)
            n1739 = call "Set pump parameters.vi"("Pump write delay (ms)"=w2647, "Volume (uL)"="Flush Center Ch Volume (uL)", "Rate (uL/h)"=w2643, "Units"=3.0, "Pump #"=2.0, "Pump Parameters In"=w2652, "VISA resource name"=w2651) -> ("Pump Parameters Out"=w2645:T47)  [unwired: 3 in]
            n1740 = Bundle By Name(cluster=w2646, "Pump 2"=w2645) -> (w2644:T10)
            n1741 = local write "All Pump Parameters"(w2644) -> ()
            n1742 = Add(x="Flush Center Ch Volume (uL)", y="Total Volume\nFlushed (uL)") -> (x+y=w2640:dbl)
            n1743 = local write "Total Volume\nFlushed (uL)"(w2640) -> ()
          }
          frame #1 {
            n1744 = Wait (ms)(milliseconds to wait=w2653) -> ()  [unwired: 1 out]
          }
          frame #2 {
            n1745 = call "Write to pump.vi"("string"="start", "VISA resource name"=w2654) -> ()  [unwired: 1 out]
          }
        }
        n1746 = local read "Save Event Log?"() -> (w2625:bool)
        n1747 = local read "Saving..."() -> (w2624:bool)
        n1748 = And(x=w2625, y=w2624) -> (x .and. y?=w2623:bool)
        n1749 = case shown="True" w2623 {
          tunnel: "Inject Pump 2" -> [_ w2634]
          frame False {
          }
          frame True {
            n1750 = local read "Flow rate (uL/h)"() -> (w2628:dbl)
            n1751 = Number To Decimal String(number=w2628) -> (decimal integer string=w2630:string)  [unwired: 1 in]
            n1752 = Concatenate Strings("on, flow rate", w2630) -> (w2629:string)
            n1753 = Select(t=w2629, s=w2634, f="off") -> (s? t:f=w2638:string)
            n1754 = local read "Time (s)"() -> (w2632:dbl)
            n1755 = local read "log file ref"() -> (w2633:refnum<file>)
            n1756 = Concatenate Strings("pump 2 ", w2638) -> (w2636:string)
            n1757 = call "write to event log.vi"("log file ref"=w2633, "time"=w2632, "input string"=w2636) -> ()  [unwired: 8 in]
          }
        }
      }
      event "Sample Channel\nFlow": Value Change {
        n1758 = event-data() -> ()  [unwired: 7 out]
        n1759 = disable-structure shown="Disabled" {
          disable-tunnel: w2656 -> [w2663 _]
          frame Disabled {
            n1760 = Select(t="irun" ("string"), s="Sample Channel\nFlow", f="stop" ("string")) -> (s? t:f=w2658:string)
            n1761 = Concatenate Strings(w2658, "\r") -> (w2661:string)
            n1762 = VISA Write(VISA resource name=w2663, write buffer=w2661) -> ()  [unwired: 1 in, 3 out]
          }
          frame Enabled {
          }
        }
      }
      event "Start Flow": Value Change {
        n1763 = event-data() -> ()  [unwired: 7 out]
        n1764 = disable-structure shown="Disabled" {
          disable-tunnel: w2664 -> [w2665 _]
          frame Disabled {
            n1765 = local write "Sample Channel\nFlow"(TRUE ("Sample Channel\nFlow")) -> ()
            n1766 = local write "Start Flow"(FALSE ("Start Flow")) -> ()
            n1767 = Concatenate Strings("irun" ("string"), "\r") -> (w2669:string)
            n1768 = VISA Write(VISA resource name=w2665, write buffer=w2669) -> ()  [unwired: 1 in, 3 out]
          }
          frame Enabled {
          }
        }
      }
      event "Stop Flow": Value Change {
        n1769 = event-data() -> ()  [unwired: 7 out]
        n1770 = disable-structure shown="Disabled" {
          disable-tunnel: w2671 -> [w2673 _]
          frame Disabled {
            w2672 = FALSE ("Stop Flow")
            n1771 = local write "Stop Flow"(w2672) -> ()
            n1772 = local write "Sample Channel\nFlow"(w2672) -> ()
            n1773 = Concatenate Strings("stop" ("string"), "\r") -> (w2675:string)
            n1774 = VISA Write(VISA resource name=w2673, write buffer=w2675) -> ()  [unwired: 1 in, 3 out]
          }
          frame Enabled {
          }
        }
      }
      event "Flow rate (uL/h)": Value Change {
        n1775 = event-data() -> ()  [unwired: 7 out]
        n1776 = disable-structure shown="Disabled" {
          disable-tunnel: w2677 -> [w2679 _]
          frame Disabled {
            n1777 = Number To Decimal String(number="Flow rate (uL/h)") -> (decimal integer string=w2683:string)  [unwired: 1 in]
            n1778 = Concatenate Strings("irate  " ("string"), w2683, " u/h" ("string"), "\r") -> (w2682:string)
            n1779 = VISA Write(VISA resource name=w2679, write buffer=w2682) -> ()  [unwired: 1 in, 3 out]
          }
          frame Enabled {
          }
        }
      }
      event "Flush Sample": Value Change {
        n1780 = event-data() -> ()  [unwired: 7 out]
        n1781 = disable-structure shown="Disabled" {
          disable-tunnel: ["Flush Sample" _] -> w2686
          disable-tunnel: w2685 -> [w2692 _]
          frame Disabled {
            n1782 = flat-sequence {
              tunnel: w2692 -> [w2733]
              tunnel: [w2713] -> w2696
              tunnel: [w2709] -> w2695
              tunnel: ["Volume (uL)"] -> w2691
              tunnel: ["Flush rate (uL/m)"] -> w2690
              tunnel: w2696 -> [w2737]
              tunnel: [w2737] -> w2694
              tunnel: w2695 -> [w2736]
              tunnel: w2694 -> [w2742]
              frame #0 {
                # "set paramaters (rate, volume) for flush, clear volume"
